vi "F8588A Test.vi"() -> ()   [LabVIEW 2020]
uses:
  DMM/3458A Digitizing Low Levels/Configure/Level Setup.ctl
  DMM/3458A Digitizing Low Levels/Configure/EXT OUT mode.ctl
  DMM/3458A Digitizing Low Levels/Configure/First Sample Trigger.ctl
  DMM/3458A Digitizing Low Levels/3458A Digitizing Low Levels.lvlib
panel:
  out "read buffer 2":string
  in  "range [V] (10V)":dbl=10.0 format="%#_13g"
  in  "stop":bool
  out "number":dbl
  out "Waveform Graph":dbl[](graph)
  in  "Reset (True)":bool
  out "error out":errorcluster
  out "read buffer":string
  in  "first sample (AUTO)":T1
  in  "samples count (100)":i32=100
  in  "EXT OUT signal (APER)":T2
  in  "LEVEL trigger":T3 caption="Cluster"
  in  "apperture [s] (1.4us)":dbl=1.4e-06 format="%#_6p"
  in  "sample period [s] (-1: use EXT trig as source)":dbl=0.0001 format="%#_6p"
  in  "VISA DMM":refnum<visa-resource-name>="GPIB0::11::INSTR"
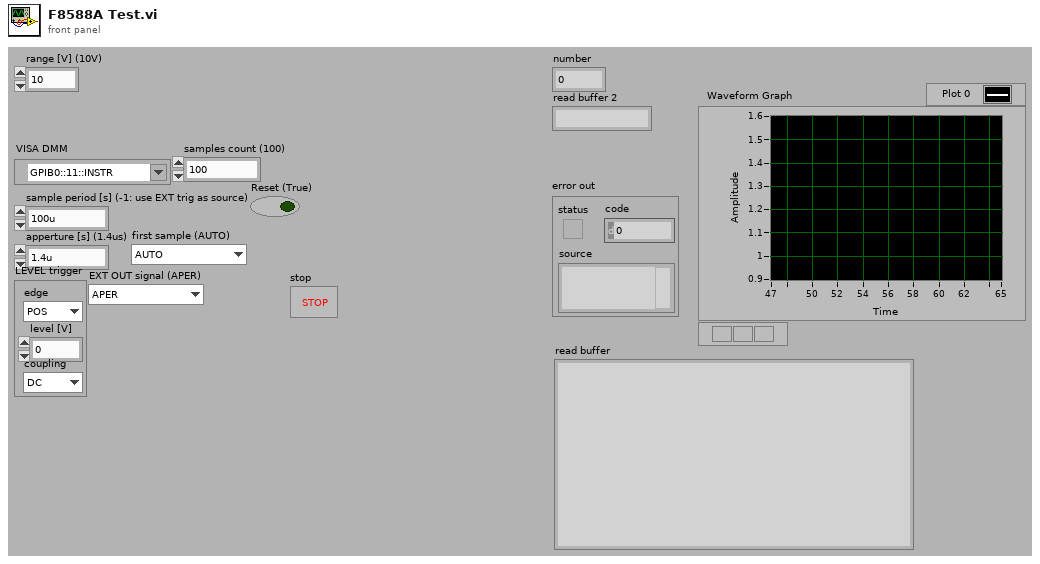
[diagram p1: front panel]
types:
  T1 = typedef "3458A Virtual Digitizer.lvlib/3458A Digitizing Low Levels.lvlib/First Sample Trigger.ctl" = enum16{"AUTO", "EXT", "SYN", "SGL", "HOLD", "LEVEL"}
  T2 = typedef "3458A Virtual Digitizer.lvlib/3458A Digitizing Low Levels.lvlib/EXT OUT mode.ctl" = enum16{"APER", "ICOMP"}
  T3 = typedef "3458A Virtual Digitizer.lvlib/3458A Digitizing Low Levels.lvlib/Level Setup.ctl" = cluster{"edge":enum16{"POS", "NEG"}, "level [V]":dbl, "coupling":enum16{"DC", "AC"}}
  T4 = enum16{"big-endian, network order", "native, host order", "little-endian"}
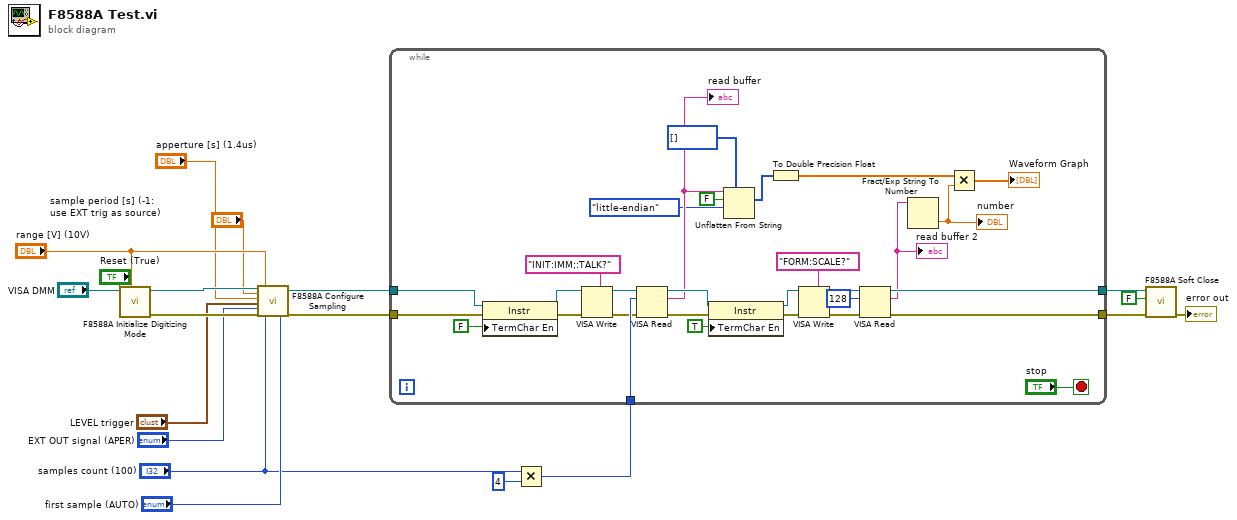
[diagram p0: block diagram]
diagram:
  n1 = call "F8588A Initialize Digitizing Mode.vi"("range [V] (10V)"="range [V] (10V)", "Reset (True)"="Reset (True)", "VISA DMM"="VISA DMM") -> ("error out"=w17:errorcluster, "VISA resource name out"=w16:refnum<visa-resource-name>)  [unwired: 5 in, 2 out]
  n2 = call "F8588A Configure Sampling.vi"("VISA resource in"=w16, "sample period [s] (-1: use EXT trig as source)"="sample period [s] (-1: use EXT trig as source)", "apperture [s] (1.4us)"="apperture [s] (1.4us)", "LEVEL trigger"="LEVEL trigger", "EXT OUT signal (APER)"="EXT OUT signal (APER)", "error in"=w17, "range [V] (10V)"="range [V] (10V)", "samples count (100)"="samples count (100)", "first sample (AUTO)"="first sample (AUTO)") -> ("VISA resource name out"=w3:refnum<visa-resource-name>, "error out"=w9:errorcluster)  [unwired: 9 in]
  n3 = Multiply(x="samples count (100)", y=4) -> (x*y=w6:i32)
  n4 = while {
    tunnel: w9 -> [w49]
    tunnel: w6 -> [w47]
    tunnel: w3 -> [w43]
    tunnel: [w31] -> w2
    tunnel: [w30] -> w1
    stop <- "stop" stop-if-true
    n5 = property class="Instr"(reference=w43, error in=w49, "TermChar En"=FALSE ("Message Based Settings:Termination Character Enable")) -> (reference out=w42:refnum<visa-resource-name>, error out=w44:errorcluster)
    n6 = VISA Write(VISA resource name=w42, write buffer="INIT:IMM;:TALK?", error in (no error)=w44) -> (VISA resource name out=w45:refnum<visa-resource-name>, error out=w46:errorcluster)  [unwired: 1 out]
    n7 = VISA Read(VISA resource name=w45, byte count=w47, error in (no error)=w46) -> (VISA resource name out=w39:refnum<visa-resource-name>, read buffer=w24:string, error out=w40:errorcluster)  [unwired: 1 out]
    "read buffer" <- w24
    n8 = property class="Instr"(reference=w39, error in=w40, "TermChar En"=TRUE ("Message Based Settings:Termination Character Enable")) -> (reference out=w36:refnum<visa-resource-name>, error out=w37:errorcluster)
    n9 = Unflatten From String(type=i32[] [], binary string=w24, data includes array or string size? (T)=FALSE, byte order (0:big-endian, network order)=T4."little-endian") -> (value=w20:i32[])  [unwired: 1 in, 2 out]
    n10 = To Double Precision Float(number=w20) -> (double precision float=w27:dbl[])
    n11 = VISA Write(VISA resource name=w36, write buffer="FORM:SCALE?", error in (no error)=w37) -> (VISA resource name out=w33:refnum<visa-resource-name>, error out=w34:errorcluster)  [unwired: 1 out]
    n12 = VISA Read(VISA resource name=w33, byte count=u32 128, error in (no error)=w34) -> (VISA resource name out=w30:refnum<visa-resource-name>, read buffer=w29:string, error out=w31:errorcluster)  [unwired: 1 out]
    "read buffer 2" <- w29
    n13 = Fract/Exp String To Number(string=w29) -> (number=w28:dbl)  [unwired: 3 in, 1 out]
    "number" <- w28
    n14 = Multiply(x=w27, y=w28) -> (x*y=→"Waveform Graph":dbl[])
  }
  n15 = call "F8588A Soft Close.vi"("error in (no error)"=w2, "Reset to preset mode (True)"=FALSE, "VISA resource name"=w1) -> ("error out"=→"error out":errorcluster)  [unwired: 8 in]
